vi "输入数据解析.vi"(0 "单个参数补充":dbl, 1 "从板号":dbl=1.0, 2 "主板二维码":string="BNET01", 3 "从板二维码":string="BNET01", 5 "主板引用":refnum<vi>, 7 "从板引用":refnum<vi>, 9 "主板选项":string="三级故障阀值", 11 "枚举":enum16{"主板", "从板"}(ring), 12 "快换":bool caption="快换写入") -> (4 "输出数组":dbl[][](array[numeric]), 6 "数组长度":dbl[](array[numeric]), 8 "循环次数":i32, 10 "命令":u32, 14 "名称":string[](array[string]), 15 "命令序号":u32[](array[numeric]))   [LabVIEW 2013] (continued)
                n2258 = call "二进制解析-8.6.vi"("索引"=4, "数值"=w5796) -> ("低位子数组"=w5794:i32[])  [unwired: 3 out]
                n2259 = disable-structure shown="启用" {
                  disable-tunnel: w5795 -> [w5805 _]
                  disable-tunnel: [w5805 255 ("高字节1")] -> w5793
                  disable-tunnel: w5794 -> [w5804 _]
                  frame Disabled {
                    (unwired) i32[] [] ("低位子数组 4")
                  }
                  frame Enabled {
                  }
                }
                n2260 = Build Array(w5793, w5793) -> (w5801:i32[])
              }
              frame 14 {
                # "内阻过大"
                n2261 = disable-structure shown="启用" {
                  disable-tunnel: w5809 -> [w5814 _]
                  disable-tunnel: [w5810 255 ("高字节1")] -> w5807
                  frame Disabled {
                    n2262 = Unbundle By Name(w5814) -> ("内阻过大"=w5813:dbl)
                    n2263 = call "输入分辨率计算-EV05.vi"("1字节?"=TRUE, "数值"=w5813, "分辨率"=0.1) -> ("高字节1"=w5810:dbl)  [unwired: 2 in, 6 out]
                  }
                  frame Enabled {
                  }
                }
                n2264 = Build Array(w5807) -> (w5808:i32[])
              }
              frame 15 {
                # "极柱温度过高"
                n2265 = disable-structure shown="启用" {
                  disable-tunnel: w5818 -> [w5824 _]
                  disable-tunnel: [w5820 255 ("高字节1")] -> w5816
                  frame Disabled {
                    n2266 = Unbundle By Name(w5824) -> ("极柱温度过高"=w5823:dbl)
                    n2267 = call "输入分辨率计算-EV05.vi"("1字节?"=TRUE, "数值"=w5823, "偏移量"=-40.0, "分辨率"=1.0) -> ("高字节1"=w5820:dbl)  [unwired: 1 in, 6 out]
                  }
                  frame Enabled {
                  }
                }
                n2268 = Build Array(w5816) -> (w5817:i32[])
              }
              frame 16 {
                # "SOH过低"
                n2269 = disable-structure shown="启用" {
                  disable-tunnel: [w5841 w5849] -> w5828
                  disable-tunnel: w5827 -> [w5838 _]
                  disable-tunnel: [w5830 w5849] -> w5826
                  frame Disabled {
                    n2270 = Unbundle By Name(w5838) -> ("SOH过低"=w5837:dbl)
                    n2271 = call "输入分辨率计算-EV05.vi"("1字节?"=FALSE, "数值"=w5837, "偏移量"=0.0, "分辨率"=0.1) -> ("低字节"=w5839:dbl, "高字节1"=w5840:dbl)  [unwired: 1 in, 5 out]
                    n2272 = call "二进制解析-8.6.vi"("索引"=4, "数值"=w5840) -> ("低位子数组"=w5843:i32[])  [unwired: 3 out]
                    n2273 = call "二进制解析-8.6.vi"("索引"=4, "数值"=w5839) -> ("低位子数组"=w5832:i32[], "高位子数组"=w5842:i32[])  [unwired: 2 out]
                    n2274 = call "二进制解析-8.6.vi"("索引"=4, "数值"=0) -> ("低位子数组"=w5833:i32[])  [unwired: 3 out]
                    n2275 = Insert Into Array(array=w5843, new element=w5842) -> (w5836:i32[])  [unwired: 1 in]
                    n2276 = Insert Into Array(array=w5832, new element=w5833) -> (w5831:i32[])  [unwired: 1 in]
                    n2277 = call "数值二进制转十进制-8.6.vi"("子数组"=w5836) -> ("十进制数值"=w5841:i32)  [unwired: 4 out]
                    n2278 = call "数值二进制转十进制-8.6.vi"("子数组"=w5831) -> ("十进制数值"=w5830:i32)  [unwired: 4 out]
                  }
                  frame Enabled {
                    w5849 = 255 ("高字节1")
                  }
                }
                n2279 = Build Array(w5828, w5826) -> (w5829:i32[])
              }
            }
            n2280 = Insert Into Array(array=w5635, new element=w5636) -> (w5634:dbl[])  [unwired: 1 in]
          }
          n2281 = Build Array(w5631) -> (w5630:dbl[][])
          n2282 = Build Array("三级故障阀值") -> (w5621:string[])
        }
        frame "单体电压过高" {
          n2283 = Unbundle By Name(w5855) -> ("一级故障"=w5856:refnum<vi>)
          n2284 = property class="Clust (严格)"(reference=w5856) -> ("Value"=w5854:T4)  [unwired: 1 in, 2 out]
          n2285 = for {
            N: 17 -> [_]
            tunnel: w5854 -> [w5866]
            shift-right: [w5863] -> w5860
            shift-left: dbl[] [] -> [w5864]
            i -> [w5867]
            n2286 = case shown="13" w5867 {
              tunnel: w5866 -> [w5868 w5879 w5890 w5900 w5910 w5920 w5932 w5944 w5956 w5968 w5980 w5992 w6006 w6027 w6039 w6048 w6057]
              tunnel: [w5869 w5880 w5891 w5901 w5911 w5922 w5934 w5946 w5958 w5970 w5982 w5993 w6015 w6030 w6038 w6047 w6059] -> w5865
              frame 0, Default {
                # "总电压过高"
                n2287 = disable-structure shown="启用" {
                  disable-tunnel: [w5875 w5878] -> w5871
                  disable-tunnel: [w5874 w5878] -> w5870
                  disable-tunnel: w5868 -> [w5873 _]
                  frame Disabled {
                    n2288 = Unbundle By Name(w5873) -> ("总电压过高"=w5872:dbl)
                    n2289 = call "输入分辨率计算-EV05.vi"("1字节?"=FALSE, "数值"=w5872, "分辨率"=0.1) -> ("低字节"=w5875:dbl, "高字节1"=w5874:dbl)  [unwired: 2 in, 5 out]
                  }
                  frame Enabled {
                    w5878 = 255 ("高字节1")
                  }
                }
                n2290 = Build Array(w5870, w5871) -> (w5869:i32[])
              }
              frame 1 {
                # "总电压过低"
                n2291 = disable-structure shown="启用" {
                  disable-tunnel: [w5886 w5889] -> w5882
                  disable-tunnel: [w5885 w5889] -> w5881
                  disable-tunnel: w5879 -> [w5884 _]
                  frame Disabled {
                    n2292 = Unbundle By Name(w5884) -> ("总电压过低"=w5883:dbl)
                    n2293 = call "输入分辨率计算-EV05.vi"("1字节?"=FALSE, "数值"=w5883, "分辨率"=0.1) -> ("低字节"=w5886:dbl, "高字节1"=w5885:dbl)  [unwired: 2 in, 5 out]
                  }
                  frame Enabled {
                    w5889 = 255 ("高字节1")
                  }
                }
                n2294 = Build Array(w5881, w5882) -> (w5880:i32[])
              }
              frame 2 {
                # "温度过高"
                n2295 = disable-structure shown="启用" {
                  disable-tunnel: [w5896 255 ("高字节1")] -> w5892
                  disable-tunnel: w5890 -> [w5894 _]
                  frame Disabled {
                    n2296 = Unbundle By Name(w5894) -> ("温度过高"=w5893:dbl)
                    n2297 = call "输入分辨率计算-EV05.vi"("1字节?"=TRUE, "数值"=w5893, "偏移量"=-40.0, "分辨率"=1.0) -> ("高字节1"=w5896:dbl)  [unwired: 1 in, 6 out]
                  }
                  frame Enabled {
                  }
                }
                n2298 = Build Array(w5892) -> (w5891:i32[])
              }
              frame 3 {
                # "温度过低"
                n2299 = disable-structure shown="启用" {
                  disable-tunnel: [w5906 255 ("高字节1")] -> w5902
                  disable-tunnel: w5900 -> [w5904 _]
                  frame Disabled {
                    n2300 = Unbundle By Name(w5904) -> ("温度过低"=w5903:dbl)
                    n2301 = call "输入分辨率计算-EV05.vi"("1字节?"=TRUE, "数值"=w5903, "偏移量"=-40.0, "分辨率"=1.0) -> ("高字节1"=w5906:dbl)  [unwired: 1 in, 6 out]
                  }
                  frame Enabled {
                  }
                }
                n2302 = Build Array(w5902) -> (w5901:i32[])
              }
              frame 4 {
                # "整组温度不均衡"
                n2303 = disable-structure shown="启用" {
                  disable-tunnel: [w5916 255 ("高字节1")] -> w5912
                  disable-tunnel: w5910 -> [w5914 _]
                  frame Disabled {
                    n2304 = Unbundle By Name(w5914) -> ("整组温度不均衡"=w5913:dbl)
                    n2305 = call "输入分辨率计算-EV05.vi"("1字节?"=TRUE, "数值"=w5913, "偏移量"=0.0, "分辨率"=1.0) -> ("高字节1"=w5916:dbl)  [unwired: 1 in, 6 out]
                  }
                  frame Enabled {
                  }
                }
                n2306 = Build Array(w5912) -> (w5911:i32[])
              }
              frame 5 {
                # "单组电压不均衡"
                n2307 = disable-structure shown="启用" {
                  disable-tunnel: [w5928 w5931] -> w5923
                  disable-tunnel: [w5926 w5931] -> w5921
                  disable-tunnel: w5920 -> [w5925 _]
                  frame Disabled {
                    n2308 = Unbundle By Name(w5925) -> ("单组电压不均衡"=w5924:dbl)
                    n2309 = call "输入分辨率计算-EV05.vi"("1字节?"=FALSE, "数值"=w5924, "偏移量"=0.0, "分辨率"=0.001) -> ("低字节"=w5926:dbl, "高字节1"=w5928:dbl)  [unwired: 1 in, 5 out]
                  }
                  frame Enabled {
                    w5931 = 255 ("高字节1")
                  }
                }
                n2310 = Build Array(w5923, w5921) -> (w5922:i32[])
              }
              frame 6 {
                # "整组电压不均衡"
                n2311 = disable-structure shown="启用" {
                  disable-tunnel: [w5940 w5943] -> w5935
                  disable-tunnel: [w5938 w5943] -> w5933
                  disable-tunnel: w5932 -> [w5937 _]
                  frame Disabled {
                    n2312 = Unbundle By Name(w5937) -> ("整组电压不均衡"=w5936:dbl)
                    n2313 = call "输入分辨率计算-EV05.vi"("1字节?"=FALSE, "数值"=w5936, "偏移量"=0.0, "分辨率"=0.001) -> ("低字节"=w5938:dbl, "高字节1"=w5940:dbl)  [unwired: 1 in, 5 out]
                  }
                  frame Enabled {
                    w5943 = 255 ("高字节1")
                  }
                }
                n2314 = Build Array(w5935, w5933) -> (w5934:i32[])
              }
              frame 7 {
                # "单体电压过高"
                n2315 = disable-structure shown="启用" {
                  disable-tunnel: [w5952 w5955] -> w5947
                  disable-tunnel: [w5950 w5955] -> w5945
                  disable-tunnel: w5944 -> [w5949 _]
                  frame Enabled {
                    n2316 = Unbundle By Name(w5949) -> ("单体电压过高"=w5948:dbl)
                    n2317 = call "输入分辨率计算-EV05.vi"("1字节?"=FALSE, "数值"=w5948, "偏移量"=0.0, "分辨率"=0.001) -> ("低字节"=w5950:dbl, "高字节1"=w5952:dbl)  [unwired: 1 in, 5 out]
                  }
                  frame Disabled {
                    w5955 = 255 ("高字节1")
                  }
                }
                n2318 = Build Array(w5947, w5945) -> (w5946:dbl[])
              }
              frame 8 {
                # "单体电压过低"
                n2319 = disable-structure shown="启用" {
                  disable-tunnel: [w5964 w5967] -> w5959
                  disable-tunnel: [w5962 w5967] -> w5957
                  disable-tunnel: w5956 -> [w5961 _]
                  frame Disabled {
                    n2320 = Unbundle By Name(w5961) -> ("单体电压过低"=w5960:dbl)
                    n2321 = call "输入分辨率计算-EV05.vi"("1字节?"=FALSE, "数值"=w5960, "偏移量"=0.0, "分辨率"=0.001) -> ("低字节"=w5962:dbl, "高字节1"=w5964:dbl)  [unwired: 1 in, 5 out]
                  }
                  frame Enabled {
                    w5967 = 255 ("高字节1")
                  }
                }
                n2322 = Build Array(w5959, w5957) -> (w5958:i32[])
              }
              frame 9 {
                # "充电电流过高"
                n2323 = disable-structure shown="启用" {
                  disable-tunnel: [w5976 w5979] -> w5971
                  disable-tunnel: [w5974 w5979] -> w5969
                  disable-tunnel: w5968 -> [w5973 _]
                  frame Disabled {
                    n2324 = Unbundle By Name(w5973) -> ("充电电流过高"=w5972:dbl)
                    n2325 = call "输入分辨率计算-EV05.vi"("1字节?"=FALSE, "数值"=w5972, "偏移量"=-3000.0, "分辨率"=0.1) -> ("低字节"=w5974:dbl, "高字节1"=w5976:dbl)  [unwired: 1 in, 5 out]
                  }
                  frame Enabled {
                    w5979 = 255 ("高字节1")
                  }
                }
                n2326 = Build Array(w5971, w5969) -> (w5970:i32[])
              }
              frame 10 {
                # "放电电流过高"
                n2327 = disable-structure shown="启用" {
                  disable-tunnel: [w5988 w5991] -> w5983
                  disable-tunnel: [w5986 w5991] -> w5981
                  disable-tunnel: w5980 -> [w5985 _]
                  frame Disabled {
                    n2328 = Unbundle By Name(w5985) -> ("放电电流过高"=w5984:dbl)
                    n2329 = call "输入分辨率计算-EV05.vi"("1字节?"=FALSE, "数值"=w5984, "偏移量"=-3000.0, "分辨率"=0.1) -> ("低字节"=w5986:dbl, "高字节1"=w5988:dbl)  [unwired: 1 in, 5 out]
                  }
                  frame Enabled {
                    w5991 = 255 ("高字节1")
                  }
                }
                n2330 = Build Array(w5983, w5981) -> (w5982:i32[])
              }
              frame 11 {
                # "单组温度不均衡"
                n2331 = disable-structure shown="启用" {
                  disable-tunnel: [w5998 255 ("高字节1")] -> w5994
                  disable-tunnel: w5992 -> [w5996 _]
                  frame Disabled {
                    n2332 = Unbundle By Name(w5996) -> ("单组温度不均衡"=w5995:dbl)
                    n2333 = call "输入分辨率计算-EV05.vi"("1字节?"=TRUE, "数值"=w5995, "偏移量"=0.0, "分辨率"=1.0) -> ("高字节1"=w5998:dbl)  [unwired: 1 in, 6 out]
                  }
                  frame Enabled {
                  }
                }
                n2334 = Build Array(w5994) -> (w5993:i32[])
              }
              frame 12 {
                # "SOC过高"
                n2335 = Unbundle By Name(w6006) -> ("SOC过高"=w6005:dbl)
                n2336 = call "输入分辨率计算-EV05.vi"("1字节?"=FALSE, "数值"=w6005, "偏移量"=0.0, "分辨率"=0.1) -> ("低字节"=w6007:dbl, "高字节1"=w6008:dbl)  [unwired: 1 in, 5 out]
                n2337 = call "二进制解析-8.6.vi"("索引"=4, "数值"=w6008) -> ("低位子数组"=w6011:i32[])  [unwired: 3 out]
                n2338 = call "二进制解析-8.6.vi"("索引"=4, "数值"=w6007) -> ("低位子数组"=w6003:i32[], "高位子数组"=w6010:i32[])  [unwired: 2 out]
                n2339 = Insert Into Array(array=w6011, new element=w6010) -> (w6009:i32[])  [unwired: 1 in]
                n2340 = call "数值二进制转十进制-8.6.vi"("子数组"=w6009) -> ("十进制数值"=w6004:i32)  [unwired: 4 out]
                n2341 = disable-structure shown="启用" {
                  disable-tunnel: w6004 -> [w6019 _]
                  disable-tunnel: [w6019 255 ("高字节1")] -> w6002
                  disable-tunnel: [w6018 i32[] [] ("低位子数组 25")] -> _
                  disable-tunnel: w6003 -> [w6018 _]
                  frame Disabled {
                  }
                  frame Enabled {
                  }
                }
                n2342 = Build Array(w6002, w6002) -> (w6015:i32[])
              }
              frame 13 {
                # "SOC过低"
                n2343 = Unbundle By Name(w6027) -> ("SOC过低"=w6026:dbl)
                n2344 = call "输入分辨率计算-EV05.vi"("1字节?"=FALSE, "数值"=w6026, "偏移量"=0.0, "分辨率"=0.1) -> ("低字节"=w6024:dbl, "高字节1"=w6025:dbl)  [unwired: 1 in, 5 out]
                n2345 = call "二进制解析-8.6.vi"("索引"=4, "数值"=w6025) -> ("低位子数组"=w6023:i32[])  [unwired: 3 out]
                n2346 = disable-structure shown="启用" {
                  disable-tunnel: w6024 -> [w6034 _]
                  disable-tunnel: [w6034 255 ("高字节1")] -> w6022
                  disable-tunnel: w6023 -> [w6033 _]
                  disable-tunnel: [w6033 i32[] [] ("低位子数组")] -> _
                  frame Disabled {
                    (unwired) i32[] [] ("低位子数组 4")
                  }
                  frame Enabled {
                  }
                }
                n2347 = Build Array(w6022, w6022) -> (w6030:i32[])
              }
              frame 14 {
                # "内阻过大"
                n2348 = disable-structure shown="启用" {
                  disable-tunnel: w6039 -> [w6044 _]
                  disable-tunnel: [w6040 255 ("高字节1")] -> w6037
                  frame Disabled {
                    n2349 = Unbundle By Name(w6044) -> ("内阻过大"=w6043:dbl)
                    n2350 = call "输入分辨率计算-EV05.vi"("1字节?"=TRUE, "数值"=w6043, "分辨率"=0.1) -> ("高字节1"=w6040:dbl)  [unwired: 2 in, 6 out]
                  }
                  frame Enabled {
                  }
                }
                n2351 = Build Array(w6037) -> (w6038:i32[])
              }
              frame 15 {
                # "极柱温度过高"
                n2352 = disable-structure shown="启用" {
                  disable-tunnel: w6048 -> [w6054 _]
                  disable-tunnel: [w6050 255 ("高字节1")] -> w6046
                  frame Disabled {
                    n2353 = Unbundle By Name(w6054) -> ("极柱温度过高"=w6053:dbl)
                    n2354 = call "输入分辨率计算-EV05.vi"("1字节?"=TRUE, "数值"=w6053, "偏移量"=-40.0, "分辨率"=1.0) -> ("高字节1"=w6050:dbl)  [unwired: 1 in, 6 out]
                  }
                  frame Enabled {
                  }
                }
                n2355 = Build Array(w6046) -> (w6047:i32[])
              }
              frame 16 {
                # "SOH过低"
                n2356 = disable-structure shown="启用" {
                  disable-tunnel: [w6071 w6079] -> w6058
                  disable-tunnel: w6057 -> [w6068 _]
                  disable-tunnel: [w6060 w6079] -> w6056
                  frame Disabled {
                    n2357 = Unbundle By Name(w6068) -> ("SOH过低"=w6067:dbl)
                    n2358 = call "输入分辨率计算-EV05.vi"("1字节?"=FALSE, "数值"=w6067, "偏移量"=0.0, "分辨率"=0.1) -> ("低字节"=w6069:dbl, "高字节1"=w6070:dbl)  [unwired: 1 in, 5 out]
                    n2359 = call "二进制解析-8.6.vi"("索引"=4, "数值"=w6070) -> ("低位子数组"=w6073:i32[])  [unwired: 3 out]
                    n2360 = call "二进制解析-8.6.vi"("索引"=4, "数值"=w6069) -> ("低位子数组"=w6062:i32[], "高位子数组"=w6072:i32[])  [unwired: 2 out]
                    n2361 = call "二进制解析-8.6.vi"("索引"=4, "数值"=0) -> ("低位子数组"=w6063:i32[])  [unwired: 3 out]
                    n2362 = Insert Into Array(array=w6073, new element=w6072) -> (w6066:i32[])  [unwired: 1 in]
                    n2363 = Insert Into Array(array=w6062, new element=w6063) -> (w6061:i32[])  [unwired: 1 in]
                    n2364 = call "数值二进制转十进制-8.6.vi"("子数组"=w6066) -> ("十进制数值"=w6071:i32)  [unwired: 4 out]
                    n2365 = call "数值二进制转十进制-8.6.vi"("子数组"=w6061) -> ("十进制数值"=w6060:i32)  [unwired: 4 out]
                  }
                  frame Enabled {
                    w6079 = 255 ("高字节1")
                  }
                }
                n2366 = Build Array(w6058, w6056) -> (w6059:i32[])
              }
            }
            n2367 = Insert Into Array(array=w5864, new element=w5865) -> (w5863:dbl[])  [unwired: 1 in]
          }
          n2368 = Build Array(w5860) -> (w5859:dbl[][])
          n2369 = Build Array("一级故障阀值") -> (w5850:string[])
        }
        frame "单体电压过高(2)" {
          n2370 = Unbundle By Name(w6085) -> ("一级故障 2"=w6086:refnum<vi>)
          n2371 = property class="Clust (严格)"(reference=w6086) -> ("Value"=w6084:T4)  [unwired: 1 in, 2 out]
          n2372 = for {
            N: 17 -> [_]
            tunnel: w6084 -> [w6096]
            shift-right: [w6093] -> w6090
            shift-left: dbl[] [] -> [w6094]
            i -> [w6097]
            n2373 = case shown="13" w6097 {
              tunnel: w6096 -> [w6098 w6109 w6120 w6130 w6140 w6150 w6162 w6174 w6186 w6198 w6210 w6222 w6236 w6257 w6269 w6278 w6287]
              tunnel: [w6099 w6110 w6121 w6131 w6141 w6152 w6164 w6176 w6188 w6200 w6212 w6223 w6245 w6260 w6268 w6277 w6289] -> w6095
              frame 0, Default {
                # "总电压过高"
                n2374 = disable-structure shown="启用" {
                  disable-tunnel: [w6105 w6108] -> w6101
                  disable-tunnel: [w6104 w6108] -> w6100
                  disable-tunnel: w6098 -> [w6103 _]
                  frame Disabled {
                    n2375 = Unbundle By Name(w6103) -> ("总电压过高"=w6102:dbl)
                    n2376 = call "输入分辨率计算-EV05.vi"("1字节?"=FALSE, "数值"=w6102, "分辨率"=0.1) -> ("低字节"=w6105:dbl, "高字节1"=w6104:dbl)  [unwired: 2 in, 5 out]
                  }
                  frame Enabled {
                    w6108 = 255 ("高字节1")
                  }
                }
                n2377 = Build Array(w6100, w6101) -> (w6099:i32[])
              }
              frame 1 {
                # "总电压过低"
                n2378 = disable-structure shown="启用" {
                  disable-tunnel: [w6116 w6119] -> w6112
                  disable-tunnel: [w6115 w6119] -> w6111
                  disable-tunnel: w6109 -> [w6114 _]
                  frame Disabled {
                    n2379 = Unbundle By Name(w6114) -> ("总电压过低"=w6113:dbl)
                    n2380 = call "输入分辨率计算-EV05.vi"("1字节?"=FALSE, "数值"=w6113, "分辨率"=0.1) -> ("低字节"=w6116:dbl, "高字节1"=w6115:dbl)  [unwired: 2 in, 5 out]
                  }
                  frame Enabled {
                    w6119 = 255 ("高字节1")
                  }
                }
                n2381 = Build Array(w6111, w6112) -> (w6110:i32[])
              }
              frame 2 {
                # "温度过高"
                n2382 = disable-structure shown="启用" {
                  disable-tunnel: [w6126 255 ("高字节1")] -> w6122
                  disable-tunnel: w6120 -> [w6124 _]
                  frame Disabled {
                    n2383 = Unbundle By Name(w6124) -> ("温度过高"=w6123:dbl)
                    n2384 = call "输入分辨率计算-EV05.vi"("1字节?"=TRUE, "数值"=w6123, "偏移量"=-40.0, "分辨率"=1.0) -> ("高字节1"=w6126:dbl)  [unwired: 1 in, 6 out]
                  }
                  frame Enabled {
                  }
                }
                n2385 = Build Array(w6122) -> (w6121:i32[])
              }
              frame 3 {
                # "温度过低"
                n2386 = disable-structure shown="启用" {
                  disable-tunnel: [w6136 255 ("高字节1")] -> w6132
                  disable-tunnel: w6130 -> [w6134 _]
                  frame Disabled {
                    n2387 = Unbundle By Name(w6134) -> ("温度过低"=w6133:dbl)
                    n2388 = call "输入分辨率计算-EV05.vi"("1字节?"=TRUE, "数值"=w6133, "偏移量"=-40.0, "分辨率"=1.0) -> ("高字节1"=w6136:dbl)  [unwired: 1 in, 6 out]
                  }
                  frame Enabled {
                  }
                }
                n2389 = Build Array(w6132) -> (w6131:i32[])
              }
              frame 4 {
                # "整组温度不均衡"
                n2390 = disable-structure shown="启用" {
                  disable-tunnel: [w6146 255 ("高字节1")] -> w6142
                  disable-tunnel: w6140 -> [w6144 _]
                  frame Disabled {
                    n2391 = Unbundle By Name(w6144) -> ("整组温度不均衡"=w6143:dbl)
                    n2392 = call "输入分辨率计算-EV05.vi"("1字节?"=TRUE, "数值"=w6143, "偏移量"=0.0, "分辨率"=1.0) -> ("高字节1"=w6146:dbl)  [unwired: 1 in, 6 out]
                  }
                  frame Enabled {
                  }
                }
                n2393 = Build Array(w6142) -> (w6141:i32[])
              }
              frame 5 {
                # "单组电压不均衡"
                n2394 = disable-structure shown="启用" {
                  disable-tunnel: [w6158 w6161] -> w6153
                  disable-tunnel: [w6156 w6161] -> w6151
                  disable-tunnel: w6150 -> [w6155 _]
                  frame Disabled {
                    n2395 = Unbundle By Name(w6155) -> ("单组电压不均衡"=w6154:dbl)
                    n2396 = call "输入分辨率计算-EV05.vi"("1字节?"=FALSE, "数值"=w6154, "偏移量"=0.0, "分辨率"=0.001) -> ("低字节"=w6156:dbl, "高字节1"=w6158:dbl)  [unwired: 1 in, 5 out]
                  }
                  frame Enabled {
                    w6161 = 255 ("高字节1")
                  }
                }
                n2397 = Build Array(w6153, w6151) -> (w6152:i32[])
              }
              frame 6 {
                # "整组电压不均衡"
                n2398 = disable-structure shown="启用" {
                  disable-tunnel: [w6170 w6173] -> w6165
                  disable-tunnel: [w6168 w6173] -> w6163
                  disable-tunnel: w6162 -> [w6167 _]
                  frame Disabled {
                    n2399 = Unbundle By Name(w6167) -> ("整组电压不均衡"=w6166:dbl)
                    n2400 = call "输入分辨率计算-EV05.vi"("1字节?"=FALSE, "数值"=w6166, "偏移量"=0.0, "分辨率"=0.001) -> ("低字节"=w6168:dbl, "高字节1"=w6170:dbl)  [unwired: 1 in, 5 out]
                  }
                  frame Enabled {
                    w6173 = 255 ("高字节1")
                  }
                }
                n2401 = Build Array(w6165, w6163) -> (w6164:i32[])
              }
              frame 7 {
                # "单体电压过高"
                n2402 = disable-structure shown="启用" {
                  disable-tunnel: [w6182 w6185] -> w6177
                  disable-tunnel: [w6180 w6185] -> w6175
                  disable-tunnel: w6174 -> [w6179 _]
                  frame Enabled {
                    n2403 = Unbundle By Name(w6179) -> ("单体电压过高"=w6178:dbl)
                    n2404 = call "输入分辨率计算-EV05.vi"("1字节?"=FALSE, "数值"=w6178, "偏移量"=0.0, "分辨率"=0.001) -> ("低字节"=w6180:dbl, "高字节1"=w6182:dbl)  [unwired: 1 in, 5 out]
                  }
                  frame Disabled {
                    w6185 = 255 ("高字节1")
                  }
                }
                n2405 = Build Array(w6177, w6175) -> (w6176:dbl[])
              }
              frame 8 {
                # "单体电压过低"
                n2406 = disable-structure shown="启用" {
                  disable-tunnel: [w6194 w6197] -> w6189
                  disable-tunnel: [w6192 w6197] -> w6187
                  disable-tunnel: w6186 -> [w6191 _]
                  frame Disabled {
                    n2407 = Unbundle By Name(w6191) -> ("单体电压过低"=w6190:dbl)
                    n2408 = call "输入分辨率计算-EV05.vi"("1字节?"=FALSE, "数值"=w6190, "偏移量"=0.0, "分辨率"=0.001) -> ("低字节"=w6192:dbl, "高字节1"=w6194:dbl)  [unwired: 1 in, 5 out]
                  }
                  frame Enabled {
                    w6197 = 255 ("高字节1")
                  }
                }
                n2409 = Build Array(w6189, w6187) -> (w6188:i32[])
              }
              frame 9 {
                # "充电电流过高"
                n2410 = disable-structure shown="启用" {
                  disable-tunnel: [w6206 w6209] -> w6201
                  disable-tunnel: [w6204 w6209] -> w6199
                  disable-tunnel: w6198 -> [w6203 _]
                  frame Disabled {
                    n2411 = Unbundle By Name(w6203) -> ("充电电流过高"=w6202:dbl)
                    n2412 = call "输入分辨率计算-EV05.vi"("1字节?"=FALSE, "数值"=w6202, "偏移量"=-3000.0, "分辨率"=0.1) -> ("低字节"=w6204:dbl, "高字节1"=w6206:dbl)  [unwired: 1 in, 5 out]
                  }
                  frame Enabled {
                    w6209 = 255 ("高字节1")
                  }
                }
                n2413 = Build Array(w6201, w6199) -> (w6200:i32[])
              }
              frame 10 {
                # "放电电流过高"
                n2414 = disable-structure shown="启用" {
                  disable-tunnel: [w6218 w6221] -> w6213
                  disable-tunnel: [w6216 w6221] -> w6211
                  disable-tunnel: w6210 -> [w6215 _]
                  frame Disabled {
                    n2415 = Unbundle By Name(w6215) -> ("放电电流过高"=w6214:dbl)
                    n2416 = call "输入分辨率计算-EV05.vi"("1字节?"=FALSE, "数值"=w6214, "偏移量"=-3000.0, "分辨率"=0.1) -> ("低字节"=w6216:dbl, "高字节1"=w6218:dbl)  [unwired: 1 in, 5 out]
                  }
                  frame Enabled {
                    w6221 = 255 ("高字节1")
                  }
                }
                n2417 = Build Array(w6213, w6211) -> (w6212:i32[])
              }
              frame 11 {
                # "单组温度不均衡"
                n2418 = disable-structure shown="启用" {
                  disable-tunnel: [w6228 255 ("高字节1")] -> w6224
                  disable-tunnel: w6222 -> [w6226 _]
                  frame Disabled {
                    n2419 = Unbundle By Name(w6226) -> ("单组温度不均衡"=w6225:dbl)
                    n2420 = call "输入分辨率计算-EV05.vi"("1字节?"=TRUE, "数值"=w6225, "偏移量"=0.0, "分辨率"=1.0) -> ("高字节1"=w6228:dbl)  [unwired: 1 in, 6 out]
                  }
                  frame Enabled {
                  }
                }
                n2421 = Build Array(w6224) -> (w6223:i32[])
              }
              frame 12 {
                # "SOC过高"
                n2422 = Unbundle By Name(w6236) -> ("SOC过高"=w6235:dbl)
                n2423 = call "输入分辨率计算-EV05.vi"("1字节?"=FALSE, "数值"=w6235, "偏移量"=0.0, "分辨率"=0.1) -> ("低字节"=w6237:dbl, "高字节1"=w6238:dbl)  [unwired: 1 in, 5 out]
                n2424 = call "二进制解析-8.6.vi"("索引"=4, "数值"=w6238) -> ("低位子数组"=w6241:i32[])  [unwired: 3 out]
                n2425 = call "二进制解析-8.6.vi"("索引"=4, "数值"=w6237) -> ("低位子数组"=w6233:i32[], "高位子数组"=w6240:i32[])  [unwired: 2 out]
                n2426 = Insert Into Array(array=w6241, new element=w6240) -> (w6239:i32[])  [unwired: 1 in]
                n2427 = call "数值二进制转十进制-8.6.vi"("子数组"=w6239) -> ("十进制数值"=w6234:i32)  [unwired: 4 out]
                n2428 = disable-structure shown="启用" {
                  disable-tunnel: w6234 -> [w6249 _]
                  disable-tunnel: [w6249 255 ("高字节1")] -> w6232
                  disable-tunnel: [w6248 i32[] [] ("低位子数组 25")] -> _
                  disable-tunnel: w6233 -> [w6248 _]
                  frame Disabled {
                  }
                  frame Enabled {
                  }
                }
                n2429 = Build Array(w6232, w6232) -> (w6245:i32[])
              }
              frame 13 {
                # "SOC过低"
                n2430 = Unbundle By Name(w6257) -> ("SOC过低"=w6256:dbl)
                n2431 = call "输入分辨率计算-EV05.vi"("1字节?"=FALSE, "数值"=w6256, "偏移量"=0.0, "分辨率"=0.1) -> ("低字节"=w6254:dbl, "高字节1"=w6255:dbl)  [unwired: 1 in, 5 out]
                n2432 = call "二进制解析-8.6.vi"("索引"=4, "数值"=w6255) -> ("低位子数组"=w6253:i32[])  [unwired: 3 out]
                n2433 = disable-structure shown="启用" {
                  disable-tunnel: w6254 -> [w6264 _]
                  disable-tunnel: [w6264 255 ("高字节1")] -> w6252
                  disable-tunnel: w6253 -> [w6263 _]
                  disable-tunnel: [w6263 i32[] [] ("低位子数组")] -> _
                  frame Disabled {
                    (unwired) i32[] [] ("低位子数组 4")
                  }
                  frame Enabled {
                  }
                }
                n2434 = Build Array(w6252, w6252) -> (w6260:i32[])
              }
              frame 14 {
                # "内阻过大"
                n2435 = disable-structure shown="启用" {
                  disable-tunnel: w6269 -> [w6274 _]
                  disable-tunnel: [w6270 255 ("高字节1")] -> w6267
                  frame Disabled {
                    n2436 = Unbundle By Name(w6274) -> ("内阻过大"=w6273:dbl)
                    n2437 = call "输入分辨率计算-EV05.vi"("1字节?"=TRUE, "数值"=w6273, "分辨率"=0.1) -> ("高字节1"=w6270:dbl)  [unwired: 2 in, 6 out]
                  }
                  frame Enabled {
                  }
                }
                n2438 = Build Array(w6267) -> (w6268:i32[])
              }
              frame 15 {
                # "极柱温度过高"
                n2439 = disable-structure shown="启用" {
                  disable-tunnel: w6278 -> [w6284 _]
                  disable-tunnel: [w6280 255 ("高字节1")] -> w6276
                  frame Disabled {
                    n2440 = Unbundle By Name(w6284) -> ("极柱温度过高"=w6283:dbl)
                    n2441 = call "输入分辨率计算-EV05.vi"("1字节?"=TRUE, "数值"=w6283, "偏移量"=-40.0, "分辨率"=1.0) -> ("高字节1"=w6280:dbl)  [unwired: 1 in, 6 out]
                  }
                  frame Enabled {
                  }
                }
                n2442 = Build Array(w6276) -> (w6277:i32[])
              }
              frame 16 {
                # "SOH过低"
                n2443 = disable-structure shown="启用" {
                  disable-tunnel: [w6301 w6309] -> w6288
                  disable-tunnel: w6287 -> [w6298 _]
                  disable-tunnel: [w6290 w6309] -> w6286
                  frame Disabled {
                    n2444 = Unbundle By Name(w6298) -> ("SOH过低"=w6297:dbl)
                    n2445 = call "输入分辨率计算-EV05.vi"("1字节?"=FALSE, "数值"=w6297, "偏移量"=0.0, "分辨率"=0.1) -> ("低字节"=w6299:dbl, "高字节1"=w6300:dbl)  [unwired: 1 in, 5 out]
                    n2446 = call "二进制解析-8.6.vi"("索引"=4, "数值"=w6300) -> ("低位子数组"=w6303:i32[])  [unwired: 3 out]
                    n2447 = call "二进制解析-8.6.vi"("索引"=4, "数值"=w6299) -> ("低位子数组"=w6292:i32[], "高位子数组"=w6302:i32[])  [unwired: 2 out]
                    n2448 = call "二进制解析-8.6.vi"("索引"=4, "数值"=0) -> ("低位子数组"=w6293:i32[])  [unwired: 3 out]
                    n2449 = Insert Into Array(array=w6303, new element=w6302) -> (w6296:i32[])  [unwired: 1 in]
                    n2450 = Insert Into Array(array=w6292, new element=w6293) -> (w6291:i32[])  [unwired: 1 in]
                    n2451 = call "数值二进制转十进制-8.6.vi"("子数组"=w6296) -> ("十进制数值"=w6301:i32)  [unwired: 4 out]
                    n2452 = call "数值二进制转十进制-8.6.vi"("子数组"=w6291) -> ("十进制数值"=w6290:i32)  [unwired: 4 out]
                  }
                  frame Enabled {
                    w6309 = 255 ("高字节1")
                  }
                }
                n2453 = Build Array(w6288, w6286) -> (w6289:i32[])
              }
            }
            n2454 = Insert Into Array(array=w6094, new element=w6095) -> (w6093:dbl[])  [unwired: 1 in]
          }
          n2455 = Build Array(w6090) -> (w6089:dbl[][])
          n2456 = Build Array("二级故障阀值") -> (w6080:string[])
        }
        frame "单体电压过高(3)" {
          n2457 = Unbundle By Name(w6315) -> ("一级故障 3"=w6316:refnum<vi>)
          n2458 = property class="Clust (严格)"(reference=w6316) -> ("Value"=w6314:T4)  [unwired: 1 in, 2 out]
          n2459 = for {
            N: 17 -> [_]
            tunnel: w6314 -> [w6326]
            shift-right: [w6323] -> w6320
            shift-left: dbl[] [] -> [w6324]
            i -> [w6327]
            n2460 = case shown="13" w6327 {
              tunnel: w6326 -> [w6328 w6339 w6350 w6360 w6370 w6380 w6392 w6404 w6416 w6428 w6440 w6452 w6466 w6487 w6499 w6508 w6517]
              tunnel: [w6329 w6340 w6351 w6361 w6371 w6382 w6394 w6406 w6418 w6430 w6442 w6453 w6475 w6490 w6498 w6507 w6519] -> w6325
              frame 0, Default {
                # "总电压过高"
                n2461 = disable-structure shown="启用" {
                  disable-tunnel: [w6335 w6338] -> w6331
                  disable-tunnel: [w6334 w6338] -> w6330
                  disable-tunnel: w6328 -> [w6333 _]
                  frame Disabled {
                    n2462 = Unbundle By Name(w6333) -> ("总电压过高"=w6332:dbl)
                    n2463 = call "输入分辨率计算-EV05.vi"("1字节?"=FALSE, "数值"=w6332, "分辨率"=0.1) -> ("低字节"=w6335:dbl, "高字节1"=w6334:dbl)  [unwired: 2 in, 5 out]
                  }
                  frame Enabled {
                    w6338 = 255 ("高字节1")
                  }
                }
                n2464 = Build Array(w6330, w6331) -> (w6329:i32[])
              }
              frame 1 {
                # "总电压过低"
                n2465 = disable-structure shown="启用" {
                  disable-tunnel: [w6346 w6349] -> w6342
                  disable-tunnel: [w6345 w6349] -> w6341
                  disable-tunnel: w6339 -> [w6344 _]
                  frame Disabled {
                    n2466 = Unbundle By Name(w6344) -> ("总电压过低"=w6343:dbl)
                    n2467 = call "输入分辨率计算-EV05.vi"("1字节?"=FALSE, "数值"=w6343, "分辨率"=0.1) -> ("低字节"=w6346:dbl, "高字节1"=w6345:dbl)  [unwired: 2 in, 5 out]
                  }
                  frame Enabled {
                    w6349 = 255 ("高字节1")
                  }
                }
                n2468 = Build Array(w6341, w6342) -> (w6340:i32[])
              }
              frame 2 {
                # "温度过高"
                n2469 = disable-structure shown="启用" {
                  disable-tunnel: [w6356 255 ("高字节1")] -> w6352
                  disable-tunnel: w6350 -> [w6354 _]
                  frame Disabled {
                    n2470 = Unbundle By Name(w6354) -> ("温度过高"=w6353:dbl)
                    n2471 = call "输入分辨率计算-EV05.vi"("1字节?"=TRUE, "数值"=w6353, "偏移量"=-40.0, "分辨率"=1.0) -> ("高字节1"=w6356:dbl)  [unwired: 1 in, 6 out]
                  }
                  frame Enabled {
                  }
                }
                n2472 = Build Array(w6352) -> (w6351:i32[])
              }
              frame 3 {
                # "温度过低"
                n2473 = disable-structure shown="启用" {
                  disable-tunnel: [w6366 255 ("高字节1")] -> w6362
                  disable-tunnel: w6360 -> [w6364 _]
                  frame Disabled {
                    n2474 = Unbundle By Name(w6364) -> ("温度过低"=w6363:dbl)
                    n2475 = call "输入分辨率计算-EV05.vi"("1字节?"=TRUE, "数值"=w6363, "偏移量"=-40.0, "分辨率"=1.0) -> ("高字节1"=w6366:dbl)  [unwired: 1 in, 6 out]
                  }
                  frame Enabled {
                  }
                }
                n2476 = Build Array(w6362) -> (w6361:i32[])
              }
              frame 4 {
                # "整组温度不均衡"
                n2477 = disable-structure shown="启用" {
                  disable-tunnel: [w6376 255 ("高字节1")] -> w6372
                  disable-tunnel: w6370 -> [w6374 _]
                  frame Disabled {
                    n2478 = Unbundle By Name(w6374) -> ("整组温度不均衡"=w6373:dbl)
                    n2479 = call "输入分辨率计算-EV05.vi"("1字节?"=TRUE, "数值"=w6373, "偏移量"=0.0, "分辨率"=1.0) -> ("高字节1"=w6376:dbl)  [unwired: 1 in, 6 out]
                  }
                  frame Enabled {
                  }
                }
                n2480 = Build Array(w6372) -> (w6371:i32[])
              }
              frame 5 {
                # "单组电压不均衡"
                n2481 = disable-structure shown="启用" {
                  disable-tunnel: [w6388 w6391] -> w6383
                  disable-tunnel: [w6386 w6391] -> w6381
                  disable-tunnel: w6380 -> [w6385 _]
                  frame Disabled {
                    n2482 = Unbundle By Name(w6385) -> ("单组电压不均衡"=w6384:dbl)
                    n2483 = call "输入分辨率计算-EV05.vi"("1字节?"=FALSE, "数值"=w6384, "偏移量"=0.0, "分辨率"=0.001) -> ("低字节"=w6386:dbl, "高字节1"=w6388:dbl)  [unwired: 1 in, 5 out]
                  }
                  frame Enabled {
                    w6391 = 255 ("高字节1")
                  }
                }
                n2484 = Build Array(w6383, w6381) -> (w6382:i32[])
              }
              frame 6 {
                # "整组电压不均衡"
                n2485 = disable-structure shown="启用" {
                  disable-tunnel: [w6400 w6403] -> w6395
                  disable-tunnel: [w6398 w6403] -> w6393
                  disable-tunnel: w6392 -> [w6397 _]
                  frame Disabled {
                    n2486 = Unbundle By Name(w6397) -> ("整组电压不均衡"=w6396:dbl)
                    n2487 = call "输入分辨率计算-EV05.vi"("1字节?"=FALSE, "数值"=w6396, "偏移量"=0.0, "分辨率"=0.001) -> ("低字节"=w6398:dbl, "高字节1"=w6400:dbl)  [unwired: 1 in, 5 out]
                  }
                  frame Enabled {
                    w6403 = 255 ("高字节1")
                  }
                }
                n2488 = Build Array(w6395, w6393) -> (w6394:i32[])
              }
              frame 7 {
                # "单体电压过高"
                n2489 = disable-structure shown="启用" {
                  disable-tunnel: [w6412 w6415] -> w6407
                  disable-tunnel: [w6410 w6415] -> w6405
                  disable-tunnel: w6404 -> [w6409 _]
                  frame Enabled {
                    n2490 = Unbundle By Name(w6409) -> ("单体电压过高"=w6408:dbl)
                    n2491 = call "输入分辨率计算-EV05.vi"("1字节?"=FALSE, "数值"=w6408, "偏移量"=0.0, "分辨率"=0.001) -> ("低字节"=w6410:dbl, "高字节1"=w6412:dbl)  [unwired: 1 in, 5 out]
                  }
                  frame Disabled {
                    w6415 = 255 ("高字节1")
                  }
                }
                n2492 = Build Array(w6407, w6405) -> (w6406:dbl[])
              }
              frame 8 {
                # "单体电压过低"
                n2493 = disable-structure shown="启用" {
                  disable-tunnel: [w6424 w6427] -> w6419
                  disable-tunnel: [w6422 w6427] -> w6417
                  disable-tunnel: w6416 -> [w6421 _]
                  frame Disabled {
                    n2494 = Unbundle By Name(w6421) -> ("单体电压过低"=w6420:dbl)
                    n2495 = call "输入分辨率计算-EV05.vi"("1字节?"=FALSE, "数值"=w6420, "偏移量"=0.0, "分辨率"=0.001) -> ("低字节"=w6422:dbl, "高字节1"=w6424:dbl)  [unwired: 1 in, 5 out]
                  }
                  frame Enabled {
                    w6427 = 255 ("高字节1")
                  }
                }
                n2496 = Build Array(w6419, w6417) -> (w6418:i32[])
              }
              frame 9 {
                # "充电电流过高"
                n2497 = disable-structure shown="启用" {
                  disable-tunnel: [w6436 w6439] -> w6431
                  disable-tunnel: [w6434 w6439] -> w6429
                  disable-tunnel: w6428 -> [w6433 _]
                  frame Disabled {
                    n2498 = Unbundle By Name(w6433) -> ("充电电流过高"=w6432:dbl)
                    n2499 = call "输入分辨率计算-EV05.vi"("1字节?"=FALSE, "数值"=w6432, "偏移量"=-3000.0, "分辨率"=0.1) -> ("低字节"=w6434:dbl, "高字节1"=w6436:dbl)  [unwired: 1 in, 5 out]
                  }
                  frame Enabled {
                    w6439 = 255 ("高字节1")
                  }
                }
                n2500 = Build Array(w6431, w6429) -> (w6430:i32[])
              }
              frame 10 {
                # "放电电流过高"
                n2501 = disable-structure shown="启用" {
                  disable-tunnel: [w6448 w6451] -> w6443
                  disable-tunnel: [w6446 w6451] -> w6441
                  disable-tunnel: w6440 -> [w6445 _]
                  frame Disabled {
                    n2502 = Unbundle By Name(w6445) -> ("放电电流过高"=w6444:dbl)
                    n2503 = call "输入分辨率计算-EV05.vi"("1字节?"=FALSE, "数值"=w6444, "偏移量"=-3000.0, "分辨率"=0.1) -> ("低字节"=w6446:dbl, "高字节1"=w6448:dbl)  [unwired: 1 in, 5 out]
                  }
                  frame Enabled {
                    w6451 = 255 ("高字节1")
                  }
                }
                n2504 = Build Array(w6443, w6441) -> (w6442:i32[])
              }
              frame 11 {
                # "单组温度不均衡"
                n2505 = disable-structure shown="启用" {
                  disable-tunnel: [w6458 255 ("高字节1")] -> w6454
                  disable-tunnel: w6452 -> [w6456 _]
                  frame Disabled {
                    n2506 = Unbundle By Name(w6456) -> ("单组温度不均衡"=w6455:dbl)
                    n2507 = call "输入分辨率计算-EV05.vi"("1字节?"=TRUE, "数值"=w6455, "偏移量"=0.0, "分辨率"=1.0) -> ("高字节1"=w6458:dbl)  [unwired: 1 in, 6 out]
                  }
                  frame Enabled {
                  }
                }
                n2508 = Build Array(w6454) -> (w6453:i32[])
              }
              frame 12 {
                # "SOC过高"
                n2509 = Unbundle By Name(w6466) -> ("SOC过高"=w6465:dbl)
                n2510 = call "输入分辨率计算-EV05.vi"("1字节?"=FALSE, "数值"=w6465, "偏移量"=0.0, "分辨率"=0.1) -> ("低字节"=w6467:dbl, "高字节1"=w6468:dbl)  [unwired: 1 in, 5 out]
                n2511 = call "二进制解析-8.6.vi"("索引"=4, "数值"=w6468) -> ("低位子数组"=w6471:i32[])  [unwired: 3 out]
                n2512 = call "二进制解析-8.6.vi"("索引"=4, "数值"=w6467) -> ("低位子数组"=w6463:i32[], "高位子数组"=w6470:i32[])  [unwired: 2 out]
                n2513 = Insert Into Array(array=w6471, new element=w6470) -> (w6469:i32[])  [unwired: 1 in]
                n2514 = call "数值二进制转十进制-8.6.vi"("子数组"=w6469) -> ("十进制数值"=w6464:i32)  [unwired: 4 out]
                n2515 = disable-structure shown="启用" {
                  disable-tunnel: w6464 -> [w6479 _]
                  disable-tunnel: [w6479 255 ("高字节1")] -> w6462
                  disable-tunnel: [w6478 i32[] [] ("低位子数组 25")] -> _
                  disable-tunnel: w6463 -> [w6478 _]
                  frame Disabled {
                  }
                  frame Enabled {
                  }
                }
                n2516 = Build Array(w6462, w6462) -> (w6475:i32[])
              }
              frame 13 {
                # "SOC过低"
                n2517 = Unbundle By Name(w6487) -> ("SOC过低"=w6486:dbl)
                n2518 = call "输入分辨率计算-EV05.vi"("1字节?"=FALSE, "数值"=w6486, "偏移量"=0.0, "分辨率"=0.1) -> ("低字节"=w6484:dbl, "高字节1"=w6485:dbl)  [unwired: 1 in, 5 out]
                n2519 = call "二进制解析-8.6.vi"("索引"=4, "数值"=w6485) -> ("低位子数组"=w6483:i32[])  [unwired: 3 out]
                n2520 = disable-structure shown="启用" {
                  disable-tunnel: w6484 -> [w6494 _]
                  disable-tunnel: [w6494 255 ("高字节1")] -> w6482
                  disable-tunnel: w6483 -> [w6493 _]
                  disable-tunnel: [w6493 i32[] [] ("低位子数组")] -> _
                  frame Disabled {
                    (unwired) i32[] [] ("低位子数组 4")
                  }
                  frame Enabled {
                  }
                }
                n2521 = Build Array(w6482, w6482) -> (w6490:i32[])
              }
              frame 14 {
                # "内阻过大"
                n2522 = disable-structure shown="启用" {
                  disable-tunnel: w6499 -> [w6504 _]
                  disable-tunnel: [w6500 255 ("高字节1")] -> w6497
                  frame Disabled {
                    n2523 = Unbundle By Name(w6504) -> ("内阻过大"=w6503:dbl)
                    n2524 = call "输入分辨率计算-EV05.vi"("1字节?"=TRUE, "数值"=w6503, "分辨率"=0.1) -> ("高字节1"=w6500:dbl)  [unwired: 2 in, 6 out]
                  }
                  frame Enabled {
                  }
                }
                n2525 = Build Array(w6497) -> (w6498:i32[])
              }
              frame 15 {
                # "极柱温度过高"
                n2526 = disable-structure shown="启用" {
                  disable-tunnel: w6508 -> [w6514 _]
                  disable-tunnel: [w6510 255 ("高字节1")] -> w6506
                  frame Disabled {
                    n2527 = Unbundle By Name(w6514) -> ("极柱温度过高"=w6513:dbl)
                    n2528 = call "输入分辨率计算-EV05.vi"("1字节?"=TRUE, "数值"=w6513, "偏移量"=-40.0, "分辨率"=1.0) -> ("高字节1"=w6510:dbl)  [unwired: 1 in, 6 out]
                  }
                  frame Enabled {
                  }
                }
                n2529 = Build Array(w6506) -> (w6507:i32[])
              }
              frame 16 {
                # "SOH过低"
                n2530 = disable-structure shown="启用" {
                  disable-tunnel: [w6531 w6539] -> w6518
                  disable-tunnel: w6517 -> [w6528 _]
                  disable-tunnel: [w6520 w6539] -> w6516
                  frame Disabled {
                    n2531 = Unbundle By Name(w6528) -> ("SOH过低"=w6527:dbl)
                    n2532 = call "输入分辨率计算-EV05.vi"("1字节?"=FALSE, "数值"=w6527, "偏移量"=0.0, "分辨率"=0.1) -> ("低字节"=w6529:dbl, "高字节1"=w6530:dbl)  [unwired: 1 in, 5 out]
                    n2533 = call "二进制解析-8.6.vi"("索引"=4, "数值"=w6530) -> ("低位子数组"=w6533:i32[])  [unwired: 3 out]
                    n2534 = call "二进制解析-8.6.vi"("索引"=4, "数值"=w6529) -> ("低位子数组"=w6522:i32[], "高位子数组"=w6532:i32[])  [unwired: 2 out]
                    n2535 = call "二进制解析-8.6.vi"("索引"=4, "数值"=0) -> ("低位子数组"=w6523:i32[])  [unwired: 3 out]
                    n2536 = Insert Into Array(array=w6533, new element=w6532) -> (w6526:i32[])  [unwired: 1 in]
                    n2537 = Insert Into Array(array=w6522, new element=w6523) -> (w6521:i32[])  [unwired: 1 in]
                    n2538 = call "数值二进制转十进制-8.6.vi"("子数组"=w6526) -> ("十进制数值"=w6531:i32)  [unwired: 4 out]
                    n2539 = call "数值二进制转十进制-8.6.vi"("子数组"=w6521) -> ("十进制数值"=w6520:i32)  [unwired: 4 out]
                  }
                  frame Enabled {
                    w6539 = 255 ("高字节1")
                  }
                }
                n2540 = Build Array(w6518, w6516) -> (w6519:i32[])
              }
            }
            n2541 = Insert Into Array(array=w6324, new element=w6325) -> (w6323:dbl[])  [unwired: 1 in]
          }
          n2542 = Build Array(w6320) -> (w6319:dbl[][])
          n2543 = Build Array("三级故障阀值") -> (w6310:string[])
        }
        frame "单体电压过低" {
          n2544 = Unbundle By Name(w6545) -> ("一级故障"=w6546:refnum<vi>)
          n2545 = property class="Clust (严格)"(reference=w6546) -> ("Value"=w6544:T4)  [unwired: 1 in, 2 out]
          n2546 = for {
            N: 17 -> [_]
            tunnel: w6544 -> [w6556]
            shift-right: [w6553] -> w6550
            shift-left: dbl[] [] -> [w6554]
            i -> [w6557]
            n2547 = case shown="13" w6557 {
              tunnel: w6556 -> [w6558 w6569 w6580 w6590 w6600 w6610 w6622 w6634 w6646 w6658 w6670 w6682 w6696 w6717 w6728 w6737 w6746]
              tunnel: [w6559 w6570 w6581 w6591 w6601 w6612 w6624 w6636 w6648 w6660 w6672 w6683 w6705 w6720 w6727 w6736 w6748] -> w6555
              frame 0, Default {
                # "总电压过高"
                n2548 = disable-structure shown="启用" {
                  disable-tunnel: [w6565 w6568] -> w6561
                  disable-tunnel: [w6564 w6568] -> w6560
                  disable-tunnel: w6558 -> [w6563 _]
                  frame Disabled {
                    n2549 = Unbundle By Name(w6563) -> ("总电压过高"=w6562:dbl)
                    n2550 = call "输入分辨率计算-EV05.vi"("1字节?"=FALSE, "数值"=w6562, "分辨率"=0.1) -> ("低字节"=w6565:dbl, "高字节1"=w6564:dbl)  [unwired: 2 in, 5 out]
                  }
                  frame Enabled {
                    w6568 = 255 ("高字节1")
                  }
                }
                n2551 = Build Array(w6560, w6561) -> (w6559:i32[])
              }
              frame 1 {
                # "总电压过低"
                n2552 = disable-structure shown="启用" {
                  disable-tunnel: [w6576 w6579] -> w6572
                  disable-tunnel: [w6575 w6579] -> w6571
                  disable-tunnel: w6569 -> [w6574 _]
                  frame Disabled {
                    n2553 = Unbundle By Name(w6574) -> ("总电压过低"=w6573:dbl)
                    n2554 = call "输入分辨率计算-EV05.vi"("1字节?"=FALSE, "数值"=w6573, "分辨率"=0.1) -> ("低字节"=w6576:dbl, "高字节1"=w6575:dbl)  [unwired: 2 in, 5 out]
                  }
                  frame Enabled {
                    w6579 = 255 ("高字节1")
                  }
                }
                n2555 = Build Array(w6571, w6572) -> (w6570:i32[])
              }
              frame 2 {
                # "温度过高"
                n2556 = disable-structure shown="启用" {
                  disable-tunnel: [w6586 255 ("高字节1")] -> w6582
                  disable-tunnel: w6580 -> [w6584 _]
                  frame Disabled {
                    n2557 = Unbundle By Name(w6584) -> ("温度过高"=w6583:dbl)
                    n2558 = call "输入分辨率计算-EV05.vi"("1字节?"=TRUE, "数值"=w6583, "偏移量"=-40.0, "分辨率"=1.0) -> ("高字节1"=w6586:dbl)  [unwired: 1 in, 6 out]
                  }
                  frame Enabled {
                  }
                }
                n2559 = Build Array(w6582) -> (w6581:i32[])
              }
              frame 3 {
                # "温度过低"
                n2560 = disable-structure shown="启用" {
                  disable-tunnel: [w6596 255 ("高字节1")] -> w6592
                  disable-tunnel: w6590 -> [w6594 _]
                  frame Disabled {
                    n2561 = Unbundle By Name(w6594) -> ("温度过低"=w6593:dbl)
                    n2562 = call "输入分辨率计算-EV05.vi"("1字节?"=TRUE, "数值"=w6593, "偏移量"=-40.0, "分辨率"=1.0) -> ("高字节1"=w6596:dbl)  [unwired: 1 in, 6 out]
                  }
                  frame Enabled {
                  }
                }
                n2563 = Build Array(w6592) -> (w6591:i32[])
              }
              frame 4 {
                # "整组温度不均衡"
                n2564 = disable-structure shown="启用" {
                  disable-tunnel: [w6606 255 ("高字节1")] -> w6602
                  disable-tunnel: w6600 -> [w6604 _]
                  frame Disabled {
                    n2565 = Unbundle By Name(w6604) -> ("整组温度不均衡"=w6603:dbl)
                    n2566 = call "输入分辨率计算-EV05.vi"("1字节?"=TRUE, "数值"=w6603, "偏移量"=0.0, "分辨率"=1.0) -> ("高字节1"=w6606:dbl)  [unwired: 1 in, 6 out]
                  }
                  frame Enabled {
                  }
                }
                n2567 = Build Array(w6602) -> (w6601:i32[])
              }
              frame 5 {
                # "单组电压不均衡"
                n2568 = disable-structure shown="启用" {
                  disable-tunnel: [w6618 w6621] -> w6613
                  disable-tunnel: [w6616 w6621] -> w6611
                  disable-tunnel: w6610 -> [w6615 _]
                  frame Disabled {
                    n2569 = Unbundle By Name(w6615) -> ("单组电压不均衡"=w6614:dbl)
                    n2570 = call "输入分辨率计算-EV05.vi"("1字节?"=FALSE, "数值"=w6614, "偏移量"=0.0, "分辨率"=0.001) -> ("低字节"=w6616:dbl, "高字节1"=w6618:dbl)  [unwired: 1 in, 5 out]
                  }
                  frame Enabled {
                    w6621 = 255 ("高字节1")
                  }
                }
                n2571 = Build Array(w6613, w6611) -> (w6612:i32[])
              }
              frame 6 {
                # "整组电压不均衡"
                n2572 = disable-structure shown="启用" {
                  disable-tunnel: [w6630 w6633] -> w6625
                  disable-tunnel: [w6628 w6633] -> w6623
                  disable-tunnel: w6622 -> [w6627 _]
                  frame Disabled {
                    n2573 = Unbundle By Name(w6627) -> ("整组电压不均衡"=w6626:dbl)
